vi "Run All Unix-compatible Expression Tests.vi"(8 "error in":errorcluster) -> (0 "error out":errorcluster)   [LabVIEW 2013]
uses:
  <vilib>/addons/_JKI Toolkits/Caraya/classes/Test/Test.lvclass
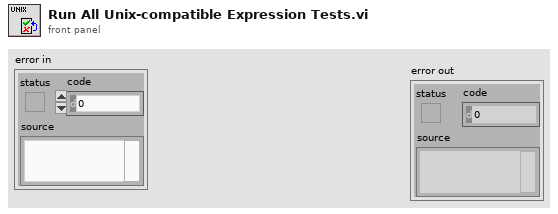
[diagram p1: front panel]
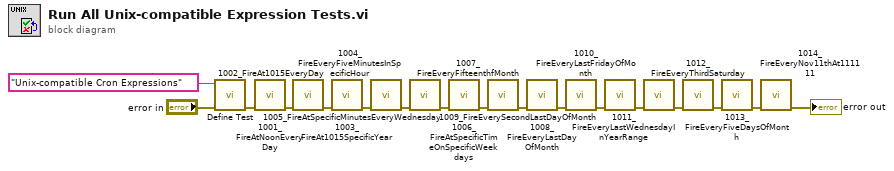
[diagram p0: block diagram]
diagram:
  n1 = call <vilib>:"Define Test.vi"("error in (no error)"="error in", "Label (VI Title)"="Unix-compatible Cron Expressions") -> ("error out"=w15:errorcluster)  [unwired: 9 in]
  n2 = call "1001_FireAtNoonEveryDay.vi"("error in (no error)"=w15) -> ("error out"=w14:errorcluster)  [unwired: 10 in]
  n3 = call "1002_FireAt1015EveryDay.vi"("error in (no error)"=w14) -> ("error out"=w13:errorcluster)  [unwired: 10 in]
  n4 = call "1003_FireAt1015SpecificYear.vi"("error in (no error)"=w13) -> ("error out"=w12:errorcluster)  [unwired: 10 in]
  n5 = call "1004_FireEveryFiveMinutesInSpecificHour.vi"("error in (no error)"=w12) -> ("error out"=w1:errorcluster)  [unwired: 10 in]
  n6 = call "1005_FireAtSpecificMinutesEveryWednesday.vi"("error in (no error)"=w1) -> ("error out"=w2:errorcluster)  [unwired: 10 in]
  n7 = call "1006_FireAtSpecificTimeOnSpecificWeekdays.vi"("error in (no error)"=w2) -> ("error out"=w3:errorcluster)  [unwired: 10 in]
  n8 = call "1007_FireEveryFifteenthfMonth.vi"("error in (no error)"=w3) -> ("error out"=w4:errorcluster)  [unwired: 10 in]
  n9 = call "1008_FireEveryLastDayOfMonth.vi"("error in (no error)"=w4) -> ("error out"=w5:errorcluster)  [unwired: 10 in]
  n10 = call "1009_FireEverySecondLastDayOfMonth.vi"("error in (no error)"=w5) -> ("error out"=w6:errorcluster)  [unwired: 10 in]
  n11 = call "1010_FireEveryLastFridayOfMonth.vi"("error in (no error)"=w6) -> ("error out"=w7:errorcluster)  [unwired: 10 in]
  n12 = call "1011_FireEveryLastWednesdayInYearRange.vi"("error in (no error)"=w7) -> ("error out"=w8:errorcluster)  [unwired: 10 in]
  n13 = call "1012_FireEveryThirdSaturday.vi"("error in (no error)"=w8) -> ("error out"=w9:errorcluster)  [unwired: 10 in]
  n14 = call "1013_FireEveryFiveDaysOfMonth.vi"("error in (no error)"=w9) -> ("error out"=w10:errorcluster)  [unwired: 10 in]
  n15 = call "1014_FireEveryNov11thAt111111.vi"("error in (no error)"=w10) -> ("error out"=→"error out":errorcluster)  [unwired: 10 in]
